vi "Build current test path.vi"(3 "error in":errorcluster) -> (7 "Current test directory":path, 10 "error out":errorcluster)   [LabVIEW 2018]
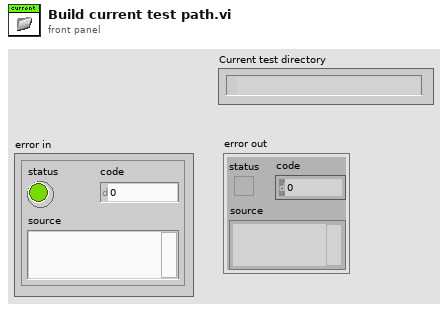
[diagram p1: front panel]
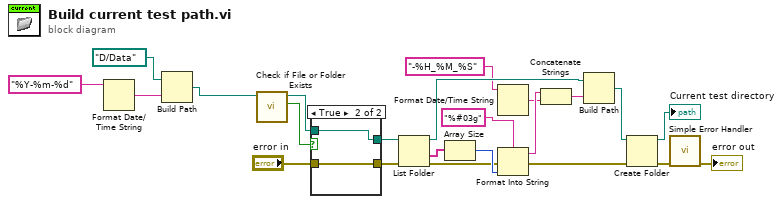
[diagram p0: block diagram]
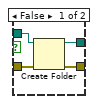
[diagram p2: hidden frame]
diagram:
  n1 = Format Date/Time String(time format string (%c)="%Y-%m-%d") -> (date/time string=w15:string)  [unwired: 2 in]
  n2 = Build Path(base path=path "D:/Data", name or relative path=w15) -> (appended path=w1:path)
  n3 = call <vilib>:"Check if File or Folder Exists.vi"("path"=w1) -> ("file or folder exists?"=w16:bool, "dup path"=w17:path)  [unwired: 8 in, 1 out]
  n4 = case shown="True" w16 {
    tunnel: w17 -> [w27 w29]
    tunnel: [w26 w29] -> w18
    tunnel: "error in" -> [w25 w28]
    tunnel: [w24 w28] -> w11
    frame False {
      n5 = Create Folder(path (use dialog)=w27, error in=w25) -> (created path=w26:path, error out=w24:errorcluster)  [unwired: 1 in, 1 out]
    }
    frame True {
    }
  }
  n6 = List Folder(path=w18, error in=w11) -> (path out=w21:path, folder names=w19:string[], error out=w10:errorcluster)  [unwired: 2 in, 1 out]
  n7 = Array Size(array=w19) -> (size(s)=w23:i32)
  n8 = Format Date/Time String(time format string (%c)="-%H_%M_%S") -> (date/time string=w3:string)  [unwired: 2 in]
  n9 = Format Into String(format string="%#03g", error in=w10, w23) -> (resulting string=w4:string, error out=w9:errorcluster)  [unwired: 1 in]
  n10 = Concatenate Strings(w4, w3) -> (w2:string)
  n11 = Build Path(base path=w21, name or relative path=w2) -> (appended path=w22:path)
  n12 = Create Folder(path (use dialog)=w22, error in=w9) -> (created path=→"Current test directory":path, error out=w8:errorcluster)  [unwired: 1 in, 1 out]
  n13 = call <vilib>:"Simple Error Handler.vi"("error in (no error)"=w8) -> ("error out"=→"error out":errorcluster)  [unwired: 4 in, 4 out]
